vi "get_temperature_waveform.vi"(9 "Config":T1={"Channel Index"=1, "Diode TC (mV)"=1.3, "Channel name"="Source-Current", "Ref voltage"=0.8, "Ref temp"=25.0} {"Ref temp" format="%.3f"; "Ref voltage" format="%.3f"; "Diode TC (mV)" format="%.3f"}, 11 "array":waveform(dbl)[](array[waveform])) -> (1 "Channel name":string, 3 "waveform out":waveform(dbl))   [LabVIEW 2019]
doc: "This example demonstrates how to acquire a continuous amount of data (Waveform) using the DAQ device's internal clock. It also shows how to synchronize two devices for different device families (E Series, S Series, M Series, X Series, DSA, and SC Express), to simultaneously acquire the data.\n\nFor instructions on how to connect your signals to the DAQ device, refer to your device documentation."
panel:
  # "Get Temperature"
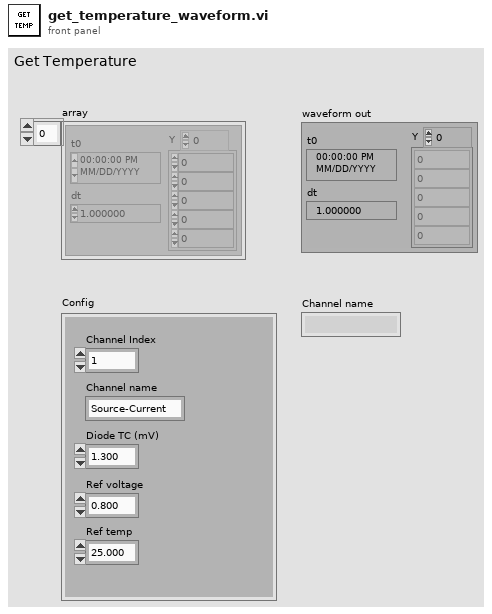
[diagram p1: front panel]
types:
  T1 = cluster{"Channel Index":i32, "Diode TC (mV)":dbl, "Channel name":string, "Ref voltage":dbl, "Ref temp":dbl}
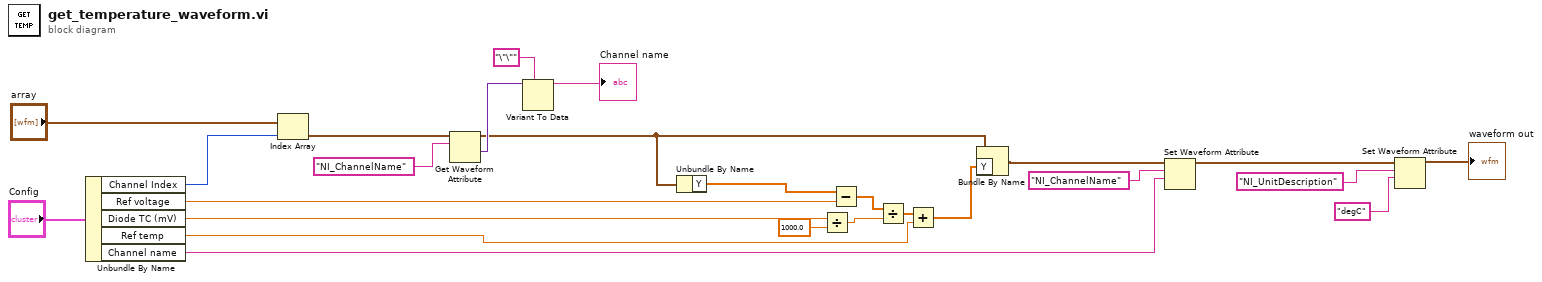
[diagram p0: block diagram]
diagram:
  n1 = Unbundle By Name("Config") -> ("Channel Index"=w16:i32, "Ref voltage"=w11:dbl, "Diode TC (mV)"=w10:dbl, "Ref temp"=w2:dbl, "Channel name"=w1:string)
  n2 = Index Array(array="array", index=w16) -> (element=w20:waveform(dbl))
  n3 = Get Waveform Attribute(6:"NI_ChannelName" ("name"), 7:w20) -> (1:w14:variant, 3:w4:waveform(dbl))  [unwired: 2 in, 2 out]
  n4 = Variant To Data(type="\"\"" ("name"), Variant=w14) -> (data=→"Channel name":string)  [unwired: 1 in, 1 out]
  n5 = Unbundle By Name(w4) -> ("Y"=w7:dbl[])
  n6 = Divide(x=w10, y=1000.0) -> (x/y=w9:dbl)
  n7 = Subtract(x=w7, y=w11) -> (x-y=w12:dbl[])
  n8 = Divide(x=w12, y=w9) -> (x/y=w6:dbl[])
  n9 = Add(x=w6, y=w2) -> (x+y=w5:dbl[])
  n10 = Bundle By Name(cluster=w4, "Y"=w5) -> (w3:waveform(dbl))
  n11 = Set Waveform Attribute(5:w1, 6:"NI_ChannelName" ("name"), 7:w3) -> (3:w22:waveform(dbl))  [unwired: 1 in, 2 out]
  n12 = Set Waveform Attribute(5:"degC" ("name"), 6:"NI_UnitDescription" ("name"), 7:w22) -> (3:→"waveform out":waveform(dbl))  [unwired: 1 in, 2 out]
